vi "updateValue.vi"(10 "Current Value in":dbl, 11 "CheckData in":refnum<class "CheckData.lvclass">) -> (3 "CheckData out":refnum<class "CheckData.lvclass">)   [LabVIEW 2017, in "CheckData.lvclass"]
uses:
  CheckData.lvclass
  CheckData.lvclass/CheckData.ctl
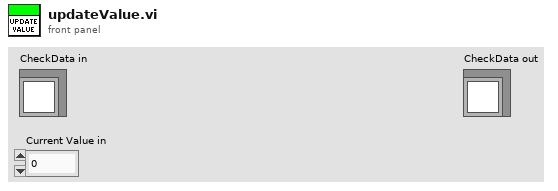
[diagram p1: front panel]
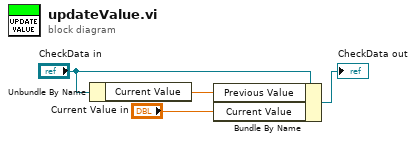
[diagram p0: block diagram]
diagram:
  n1 = Unbundle By Name("CheckData in") -> ("Current Value"=w2:dbl)
  n2 = Bundle By Name(cluster="CheckData in", "Previous Value"=w2, "Current Value"="Current Value in") -> (→"CheckData out":refnum<class "CheckData.lvclass">)
